vi "Hot or Not.vi"() -> (1 "HotOrNot":bool)   [LabVIEW 2013]
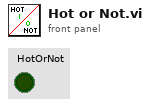
[diagram p1: front panel]
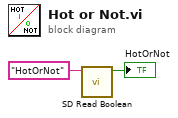
[diagram p0: block diagram]
diagram:
  n1 = call <vilib>:"SD Read Boolean.vi"("Name"="HotOrNot") -> ("Boolean"=→"HotOrNot":bool)  [unwired: 8 in, 2 out]
